vi "ReadAppKeyFile.vi"(7 "Task":enum16{"Read", "Write"}(ring), 8 "error in (no error)":errorcluster, 11 "Device In":T1={"Name"="", "BaseURL"="", "AppKey"="", "Headers"=["Content-Type:application/json"], "Timeout"=10000}) -> (0 "error out":errorcluster, 2 "text":string, 3 "Device Out":T1={"Name"="", "BaseURL"="", "AppKey"="", "Headers"=["Content-Type:application/json"], "Timeout"=10000})   [LabVIEW 2019]
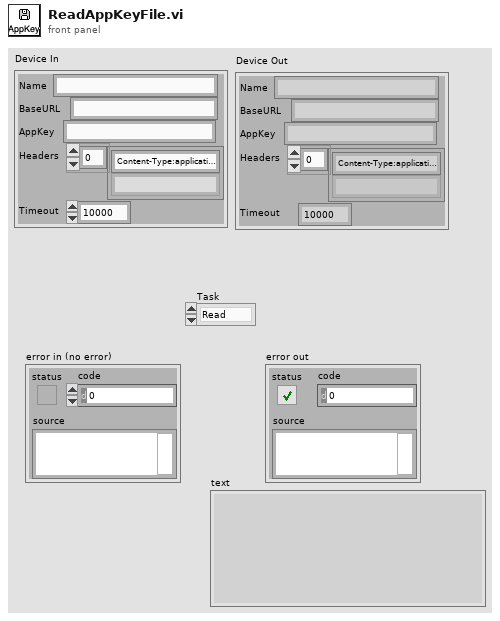
[diagram p1: front panel]
types:
  T1 = cluster{"Name":string, "BaseURL":string, "AppKey":string, "Headers":string[], "Timeout":i32}
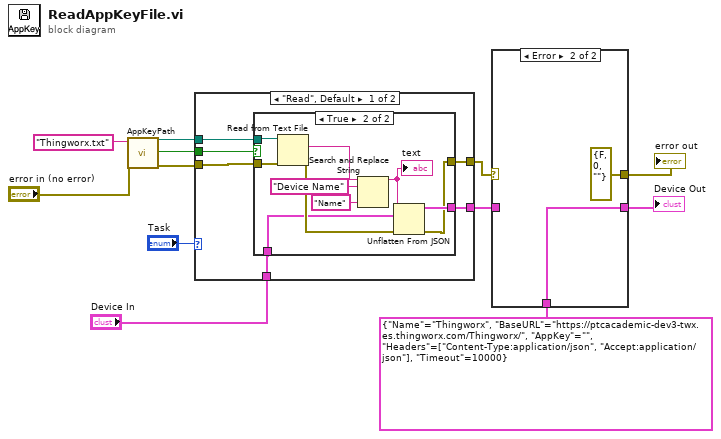
[diagram p0: block diagram]
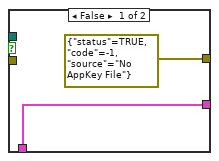
[diagram p3: hidden frame]
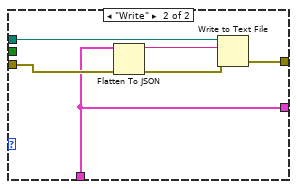
[diagram p4: hidden frame]
diagram:
  n1 = call "AppKeyPath.vi"("error in (no error)"="error in (no error)", "FileName"="Thingworx.txt" ("Name")) -> ("error out"=w3:errorcluster, "exists?"=w4:bool, "AppKeyPath"=w5:path)  [unwired: 7 in]
  n2 = case shown="\"Read\", Default" "Task" {
    tunnel: w5 -> [w17 w36]
    tunnel: w3 -> [w18 w34]
    tunnel: [w16 w32] -> w10
    tunnel: w4 -> [w15 _]
    tunnel: [w14 w31] -> w9
    tunnel: "Device In" -> [w13 w31]
    frame "Read", Default {
      n3 = case shown="True" w15 {
        tunnel: w18 -> [_ w30]
        tunnel: w17 -> [_ w29]
        tunnel: [errorcluster {"status"=TRUE, "code"=-1, "source"="No AppKey File"} ("error out") w25] -> w16
        tunnel: [w19 w26] -> w14
        tunnel: w13 -> [w19 w27]
        frame False {
        }
        frame True {
          n4 = Read from Text File(file (use dialog)=w29, error in=w30) -> (text=w24:string, error out=w28:errorcluster)  [unwired: 2 in, 2 out]
          n5 = Search and Replace String(input string=w24, search string="Device Name", replace string="Name" ("replace string (\"\")")) -> (result string=w21:string)  [unwired: 5 in, 3 out]
          "text" <- w21
          n6 = Unflatten From JSON(JSON string=w21, type and defaults=w27, error in (no error)=w28) -> (value=w26:T1, error out=w25:errorcluster)  [unwired: 4 in]
        }
      }
    }
    frame "Write" {
      n7 = Flatten To JSON(anything=w31, error in (no error)=w34) -> (JSON string=w35:string, 11:w33:errorcluster)  [unwired: 1 in]
      n8 = Write to Text File(file (use dialog)=w36, text=w35, error in=w33) -> (error out=w32:errorcluster)  [unwired: 1 in, 2 out]
    }
  }
  n9 = case shown="Error" w10 {
    selector: w10 -> [w37 _]
    tunnel: [w38 w39] -> w6
    tunnel: w9 -> [w38 _]
    tunnel: [w37 errorcluster {"status"=FALSE, "code"=0, "source"=""} ("error IO")] -> w8
    tunnel: T1 {"Name"="Thingworx", "BaseURL"="https://ptcacademic-dev3-twx.es.thingworx.com/Thingworx/", "AppKey"="", "Headers"=["Content-Type:application/json", "Accept:application/json"], "Timeout"=10000} ("Device In") -> [_ w39]
    frame No Error {
    }
    frame Error {
    }
  }
  "error out" <- w8
  "Device Out" <- w6
